vi "打开excel.vi"(8 "错误输入（无错误）":errorcluster, 10 "excel路径":path, 11 "工作簿引用":refnum<k7>) -> (0 "错误输出":errorcluster, 2 "excel引用":refnum<k7>, 3 "工作簿输出":refnum<k7>)   [LabVIEW 2013, in "excel处理.lvlib"]
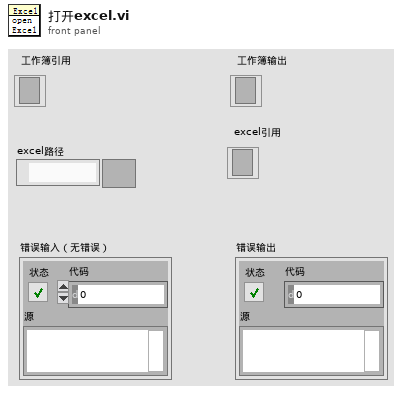
[diagram p1: front panel]
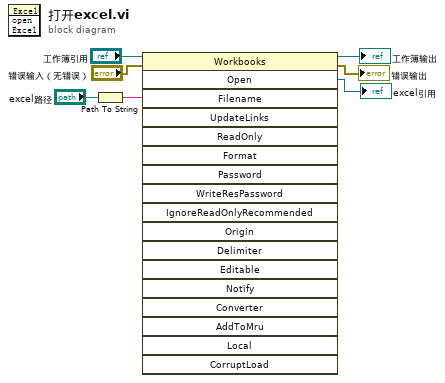
[diagram p0: block diagram]
diagram:
  n1 = Path To String(path="excel路径") -> (string=w7:string)
  n2 = invoke on="调用节点" class="Workbooks" method="Open"(reference="工作簿引用", error in="错误输入（无错误）", "Filename"=w7) -> (reference out=→"工作簿输出":refnum<k7>, error out=→"错误输出":errorcluster, "Open"=→"excel引用":refnum<k7>)  [unwired: 15 in, 15 out]
